vi "RT_AIChar_v2.vi"() -> ()   [LabVIEW 2020]
uses:
  <vilib>/rvi/interface/nirviReadWriteControl/nirviReadWriteControl.xnode
  <vilib>/Platform/TimedLoop/XDataNode/XDataNode.xnode
  <vilib>/Platform/TimedLoop/XDataNode/nitl_modes.ctl
  <vilib>/Platform/TimedLoop/XDataNode/XDNodeRunTimeDep.lvlib
  <vilib>/Platform/TimedLoop/XDataNode/wakeup.ctl
  <vilib>/Platform/TimedLoop/XDataNode/timing_clust.ctl
  Components_global/Timing/Timing.lvlib
  <vilib>/rvi/interface/nirviOpenFPGA/nirviOpenFPGA.xnode
  <vilib>/NI/STM/NI STM.lvlib
  <vilib>/NI/STM/SubVIs/MetaDataElement.ctl
  <vilib>/NI/STM/TCP/Write Message (TCP).vi
  <vilib>/rvi/interface/Simulation/niFpgaSimulationCallBeginRW.vi
  <vilib>/rvi/errors/niLvFpgaAdjustHostInterfaceError.vi
  <vilib>/rvi/interface/nirviCloseFPGA/nirviCloseFPGA.xnode
  NiFpgaLv.dll
  <vilib>/Utility/error.llb/Error Cluster From Error Code.vi
  <vilib>/NI/STM/TCP/Get Connection Reference (TCP).vi
  <vilib>/NI/STM/TCP/Write Meta Data (TCP Ref).vi
  <vilib>/FPGAPlugInAG/Dynamic/niLvFpga_Close_Dynamic.vi
  FPGA Bitfiles/levitationcode_FPGATarget_FPGAmainIOtestv3_bLcpaLDc0zo.lvbitx
  FPGA/AIchar/FPGA_main_IOtest_v4.vi
  <vilib>/FPGAPlugInAG/cRIO-9049/niLvFpga_Open_cRIO-9049.vi
  <vilib>/rvi/interface/common/dynamic/niFpgaDynamicAddResources.vi
  FPGA/Components/FPGA TypeDefs/SelectAOchannel_Enum.ctl
panel:
  in  "Select AO channel":T1
  in  "Excitation mode":T2(ring)
  in  "Frequency [Hz]":dbl
  in  "Amplitude [V]":dbl
  in  "Select channel":T3(ring)
  in  "Select Module":T4(ring)
  out "RT Loop Rate":dbl format="%.3p"
  out "# of iterations\n[STM write]":i32
  out "# elements \nFIFO buffer":u32
  out "Finished \nlate counter?":dbl
  in  "stop":bool
  # "Analog Ouput"
  # "- Open PC_SensorChar vi and run that VI as well to start capturing data!"
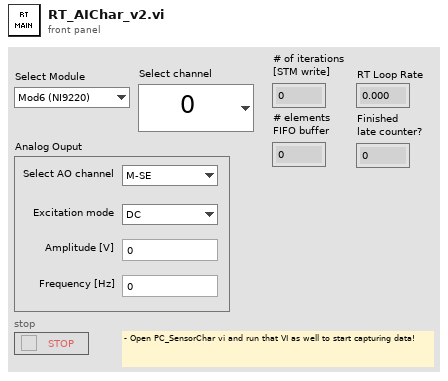
[diagram p1: front panel]
types:
  T1 = typedef "SelectAOchannel_Enum.ctl" = enum8{"M-SE", "M-NE", "M-NW", "M-SW", "M-CO", "M-CI"}
  T2 = enum16{"DC", "Sinewave", "Squarewave", "WhiteNoise"}
  T3 = enum16{"0", "1", "2", "3", "4", "5", "6", "7", "8", "9", "10", "11", "12", "13", "14", "15"}
  T4 = enum16{"Mod6 (NI9220)", "Mod7 (NI9220)", "Mod8 (NI9222)"}
  T5 = typedef "NI STM.lvlib/MetaDataElement.ctl" = string
  T6 = typedef "NI STM.lvlib/TCP Connection Info.ctl" = cluster{"connection ID":refnum<k5>, "meta data":T5[]}
  T7 = typedef "XDNodeRunTimeDep.lvlib/timing_clust.ctl" = cluster{"Expected End [f-1]":u64, "Actual End [f-1]":u64, "Finished Late? [f-1]":bool, "Expected End [i-1]":u64, "Actual End [i-1]":u64, "Finished Late? [i-1]":bool, "Expected Start [i]":u64, "Actual Start [i]":u64, "Expected Start [f]":u64, "Actual Start [f]":u64, "Source Name":string, "Structure Name":string, "Period":i64, "Deadline":i64, "Offset":i64, "Start":i64, "Priority":i32, "Timeout":i32, "Mode":T8, "Wakeup Reason":T9, "Error":errorcluster, "Source Type":string, "Secondary Source Type":string, "Global End Time":u64, "Global Start Time":u64, "Frame Duration":u64, "Iteration Duration":u64, "Assigned CPU":i32, "I/O Scan Engine Mode":u32}
  T8 = typedef "XDNodeRunTimeDep.lvlib/nitl_modes.ctl" = enum32{"No Change", "Process missed periods, maintain original phase", "Discard missed periods, maintain original phase", "Process missed periods, ignore original phase", "Discard missed periods, ignore original phase"}
  T9 = typedef "XDNodeRunTimeDep.lvlib/wakeup.ctl" = enum32{"Normal", "Aborted", "Asynchronous wakeup", "Timing source error", "Timed loop error", "Timeout"}
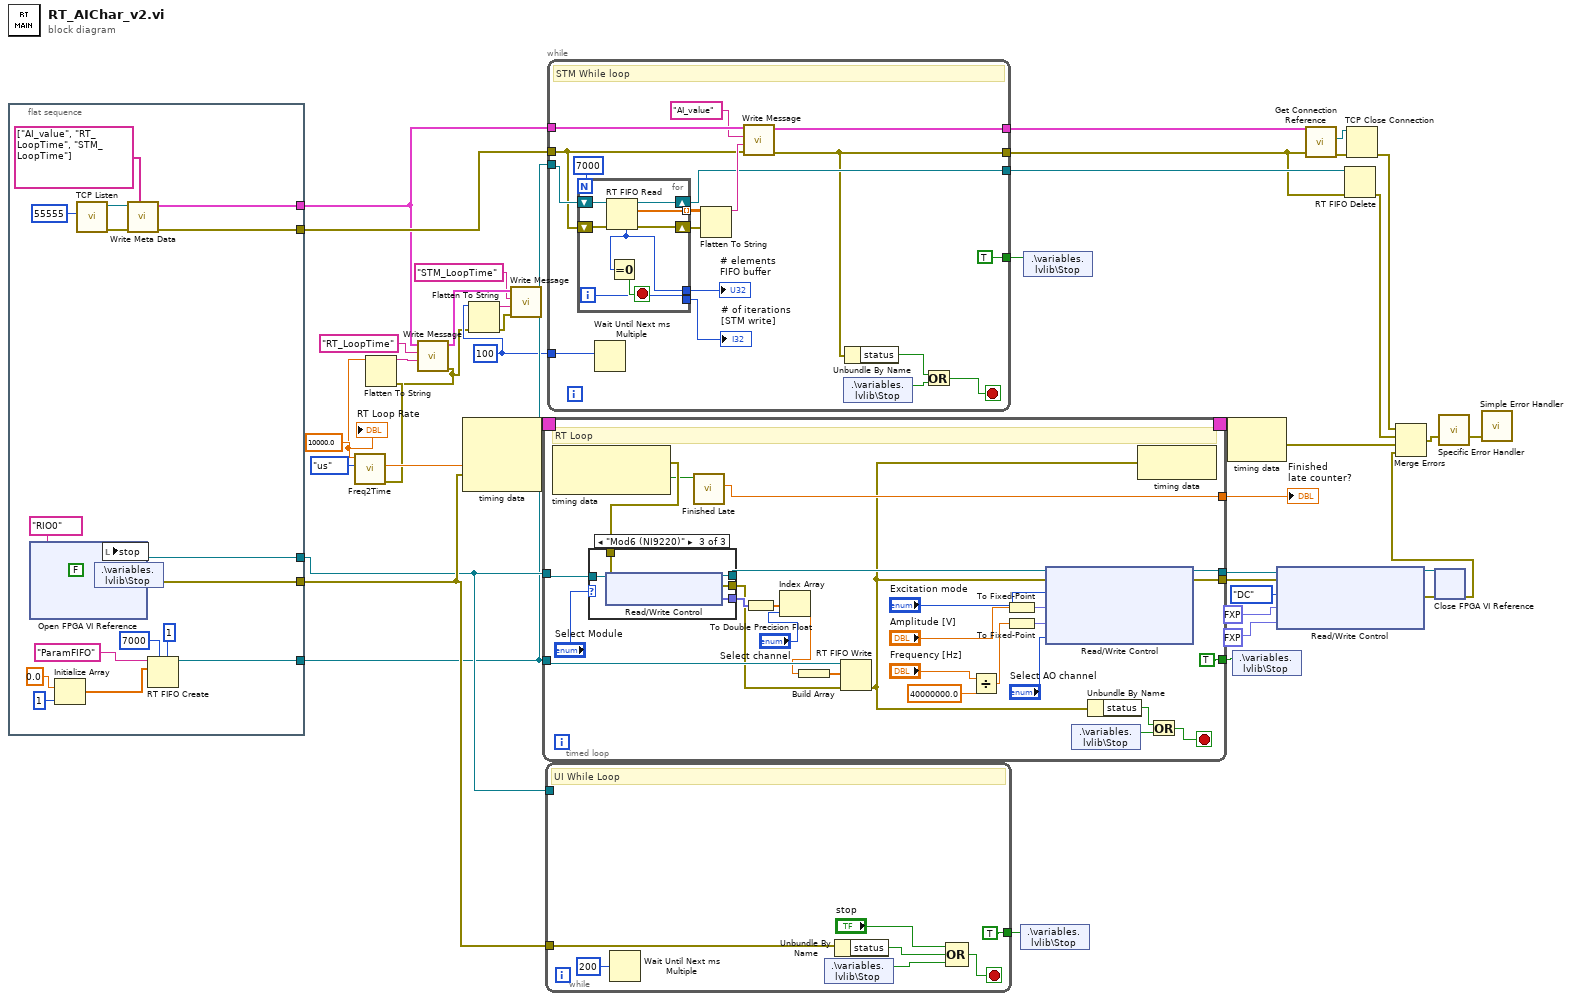
[diagram p0: block diagram]
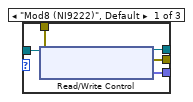
[diagram p2: hidden frame]
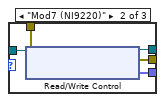
[diagram p3: hidden frame]
diagram:
  w7 = u32 100 ("millisecond multiple")
  n1 = flat-sequence {
    tunnel: [w58] -> w21
    tunnel: [w57] -> w20
    tunnel: [w52] -> w4
    tunnel: [w51] -> w36
    tunnel: [w50] -> w8
    frame #0 {
      w59 = FALSE ("Stop")
      n2 = xnode "Open FPGA VI Reference"("resource name"=tag "RIO0") -> ("FPGA VI Reference Out"=w57:refnum<k20>, "error out"=w60:errorcluster)  [unwired: 1 in]
      n3 = Initialize Array(0.0 ("element"), 1 ("dimension size")) -> (w45:dbl[])
      n4 = call <vilib>:"TCP Listen.vi"("port"=u16 55555) -> ("error out"=w55:errorcluster, "connection ID"=w54:refnum<k5>)  [unwired: 6 in, 3 out]
      n5 = shared-variable ".\\variables.lvlib\\Stop"(w59, error in=w60) -> (error out=w58:errorcluster)
      n6 = local write "stop"(w59) -> ()
      n7 = call-poly <vilib>:"Write Meta Data.vi"("meta data"=T5[] ["AI_value", "RT_LoopTime", "STM_LoopTime"], "error in"=w55, "connection ID"=w54) -> ("error out"=w51:errorcluster, "connection info out"=w52:T6)  [unwired: 7 in]
      n8 = RT FIFO Create(0:"ParamFIFO" ("name (unnamed)"), 1:w45, 4:u32 7000 ("size (10)"), 6:u32 1 ("elements in array (1)")) -> (8:w50:refnum<k33>)  [unwired: 4 in, 2 out]
    }
  }
  n9 = call "Freq2Time.vi"("Int. Time Unit"=enum16{"sec", "us", "ms"}."us", "Sample rate (Hz)"=10000.0 ("Period")) -> ("error out"=w25:errorcluster, "Int.  time [unit]"=w37:dbl, "New Sample rate (Hz)"=w27:dbl)  [unwired: 7 in]
  "RT Loop Rate" <- w27
  n10 = Flatten To String(anything=w27, error in (no error)=w25) -> (data string=w28:string, error out=w6:errorcluster)  [unwired: 2 in, 1 out]
  n11 = call-poly <vilib>:"Write Message.vi"("error in"=w6, "data"=w28, "name"="RT_LoopTime", "connection info in"=w4) -> ("connection info out"=w3:T6)  [unwired: 6 in, 1 out]
  n12 = node-c288(w37, w21) -> (w42:T7)  [unwired: 1 in]
  n13 = Flatten To String(anything=w7, error in (no error)=w6) -> (data string=w1:string, error out=w5:errorcluster)  [unwired: 2 in, 1 out]
  n14 = call-poly <vilib>:"Write Message.vi"("error in"=w5, "data"=w1, "name"="STM_LoopTime", "connection info in"=w3) -> ()  [unwired: 6 in, 2 out]
  n15 = timed-loop {
    tunnel: w20 -> [w88]
    timing: w42 -> [_]
    timing-out: [_] -> w41
    tunnel: [w85] -> w40
    tunnel: w8 -> [w84]
    tunnel: [TRUE ("Stop")] -> w10
    tunnel: [w71] -> w18
    tunnel: [w70] -> w16
    stop <- w82 stop-if-true
    # "RT Loop"
    n16 = node-c288() -> (w87:errorcluster, w86:bool)  [unwired: 1 in]
    n17 = case shown="\"Mod6 (NI9220)\"" "Select Module" {
      tunnel: w88 -> [w93 w98 w103]
      tunnel: w87 -> [w92 w97 w102]
      tunnel: [w91 w96 w101] -> w75
      tunnel: [w90 w95 w100] -> w72
      tunnel: [w89 w94 w99] -> w74
      frame "Mod8 (NI9222)", Default {
        n18 = xnode "Read/Write Control"("FPGA VI Reference In"=w93, "error in"=w92) -> ("FPGA VI Reference Out"=w90:refnum<k20>, "error out"=w89:errorcluster, "Mod8 (NI 9222) AI"=w91:fxp<+/-,25,5>[])
      }
      frame "Mod7 (NI9220)" {
        n19 = xnode "Read/Write Control"("FPGA VI Reference In"=w98, "error in"=w97) -> ("FPGA VI Reference Out"=w95:refnum<k20>, "error out"=w94:errorcluster, "Mod7 (NI 9222) AI"=w96:fxp<+/-,25,5>[])
      }
      frame "Mod6 (NI9220)" {
        n20 = xnode "Read/Write Control"("FPGA VI Reference In"=w103, "error in"=w102) -> ("FPGA VI Reference Out"=w100:refnum<k20>, "error out"=w99:errorcluster, "Mod6 (NI 9222) AI"=w101:fxp<+/-,25,5>[])
      }
    }
    n21 = call "Finished Late.vi"("Finished \nLate?"=w86) -> ("# Finished\nLate counter"=w85:dbl)  [unwired: 8 in, 2 out]
    n22 = To Double Precision Float(number=w75) -> (double precision float=w79:dbl[])
    n23 = Index Array(array=w79, index="Select channel") -> (element=w77:dbl)
    n24 = Build Array(w77) -> (w78:dbl[])
    n25 = RT FIFO Write(0:w84, 1:w78, 3:w74) -> (11:w69:errorcluster)  [unwired: 2 in, 3 out]
    n26 = Divide(x="Frequency [Hz]", y=40000000.0) -> (x/y=w65:dbl)
    n27 = To Fixed-Point(number="Amplitude [V]") -> (fixed-point=w64:fxp<+/-,16,5>)  [unwired: 1 in]
    n28 = To Fixed-Point(number=w65) -> (fixed-point=w66:fxp<+,32,0>)  [unwired: 1 in]
    n29 = xnode "Read/Write Control"("FPGA VI Reference In"=w72, "error in"=w69, "Excitation mode"="Excitation mode", "Amplitude [V]"=w64, "Frequency [periods/tick]"=w66, "Select AO channel"="Select AO channel") -> ("FPGA VI Reference Out"=w71:refnum<k20>, "error out"=w70:errorcluster)
    n30 = shared-variable ".\\variables.lvlib\\Stop"() -> (w81:bool)  [unwired: 1 in, 1 out]
    n31 = Unbundle By Name(w69) -> ("status"=w80:bool)
    n32 = node-c288(w69) -> ()  [unwired: 1 out]
    n33 = Or(x=w80, y=w81) -> (x .or. y?=w82:bool)
  }
  "Finished \nlate counter?" <- w40
  n34 = while {
    tunnel: w21 -> [w112]
    tunnel: w20 -> [_]
    tunnel: [TRUE ("Stop")] -> w9
    stop <- w113 stop-if-true
    # "UI While Loop"
    n35 = Wait Until Next ms Multiple(millisecond multiple=u32 200) -> ()  [unwired: 1 out]
    n36 = shared-variable ".\\variables.lvlib\\Stop"() -> (w114:bool)  [unwired: 1 in, 1 out]
    n37 = Unbundle By Name(w112) -> ("status"=w111:bool)
    n38 = Compound Arithmetic op=OR("stop", w111, w114) -> (w113:bool)
  }
  n39 = while {
    tunnel: w4 -> [w134]
    tunnel: w36 -> [w128]
    tunnel: [w132] -> w35
    tunnel: [w118] -> w31
    tunnel: w8 -> [w130]
    tunnel: [w127] -> w32
    tunnel: [TRUE ("Stop")] -> w11
    tunnel: w7 -> [w117]
    stop <- w120 stop-if-true
    # "STM While loop"
    n40 = for {
      N: 7000 -> [_]
      shift-right: [w139] -> w127
      shift-left: w130 -> [w142]
      shift-right: [w141] -> w129
      shift-left: w128 -> [w140]
      tunnel: [w138] -> w126
      tunnel: [w136] -> w125
      tunnel: [w135] -> w124 mode=indexing
      i -> [w136]
      stop <- w137 stop-if-true
      n41 = RT FIFO Read(0:w142, 3:w140) -> (7:w138:u32, 8:w139:refnum<k33>, 9:w135:dbl[], 11:w141:errorcluster)  [unwired: 2 in, 1 out]
      n42 = Equal To 0?(x=w138) -> (x = 0?=w137:bool)
    }
    "# elements \nFIFO buffer" <- w126
    "# of iterations\n[STM write]" <- w125
    n43 = Wait Until Next ms Multiple(millisecond multiple=w117) -> ()  [unwired: 1 out]
    n44 = Flatten To String(anything=w124, error in (no error)=w129) -> (data string=w131:string)  [unwired: 2 in, 2 out]
    n45 = call-poly <vilib>:"Write Message.vi"("error in"=w128, "data"=w131, "name"="AI_value", "connection info in"=w134) -> ("error out"=w118:errorcluster, "connection info out"=w132:T6)  [unwired: 6 in]
    n46 = shared-variable ".\\variables.lvlib\\Stop"() -> (w121:bool)  [unwired: 1 in, 1 out]
    n47 = Unbundle By Name(w118) -> ("status"=w119:bool)
    n48 = Or(x=w119, y=w121) -> (x .or. y?=w120:bool)
  }
  n49 = shared-variable ".\\variables.lvlib\\Stop"(w9) -> ()  [unwired: 1 in, 1 out]
  n50 = shared-variable ".\\variables.lvlib\\Stop"(w11) -> ()  [unwired: 1 in, 1 out]
  n51 = node-c288(w41) -> (w26:errorcluster)
  n52 = shared-variable ".\\variables.lvlib\\Stop"(w10) -> ()  [unwired: 1 in, 1 out]
  n53 = xnode "Read/Write Control"("FPGA VI Reference In"=w18, "error in"=w16, "Excitation mode"=T2."DC", "Amplitude [V]"=fxp<+/-,16,5> 0.0, "Frequency [periods/tick]"=fxp<+,32,0> 0.0) -> ("FPGA VI Reference Out"=w17:refnum<k20>, "error out"=w15:errorcluster)
  n54 = call-poly <vilib>:"Get Connection Reference.vi"("error in"=w31, "connection info in"=w35) -> ("error out"=w34:errorcluster, "connection ID out"=w33:refnum<k5>)  [unwired: 7 in, 1 out]
  n55 = RT FIFO Delete(0:w32, 3:w31) -> (11:w30:errorcluster)  [unwired: 1 in]
  n56 = TCP Close Connection(connection ID=w33, error in (no error)=w34) -> (error out=w22:errorcluster)  [unwired: 1 in, 1 out]
  n57 = xnode "Close FPGA VI Reference"("FPGA VI Reference In"=w17, "error in"=w15) -> ("error out"=w19:errorcluster)
  n58 = Merge Errors(w22, w30, w26, w19) -> (w24:errorcluster)
  n59 = call "Specific Error Handler"("Error to Check"=w24) -> ("error out"=w23:errorcluster)  [unwired: 11 in, 3 out]
  n60 = call <vilib>:"Simple Error Handler.vi"("error in (no error)"=w23) -> ()  [unwired: 4 in, 5 out]
